vi "Write to DB.vi"() -> ()   [LabVIEW 2017]
uses:
  Type Definitions/DB Record.ctl
panel:
  in  "DB Record":T1 {"Balance" format="%.2f"; "Account" format="%05d"}
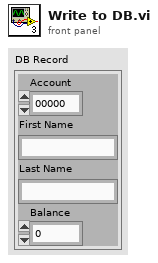
[diagram p1: front panel]
types:
  T1 = typedef "DB Record.ctl" = cluster{"Account":i32, "First Name":string, "Last Name":string, "Balance":fxp<+/-,64,35>}
  T2 = enum16{"open", "replace", "create", "open or create", "replace or create", "replace or create with confirmation"}
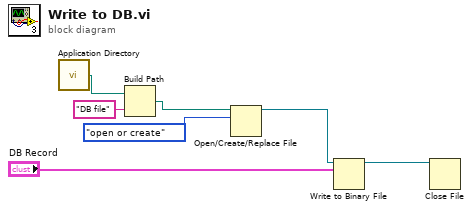
[diagram p0: block diagram]
diagram:
  n1 = call <vilib>:"Application Directory.vi"() -> ("Application Directory"=w1:path)
  n2 = Build Path(base path=w1, name or relative path="DB file") -> (appended path=w3:path)
  n3 = Open/Create/Replace File(file path (use dialog)=w3, operation (0:open)=T2."open or create") -> (refnum out=w7:refnum<file>)  [unwired: 4 in, 2 out]
  n4 = Write to Binary File(file (use dialog)=w7, data="DB Record") -> (refnum out=w5:refnum<file>)  [unwired: 4 in, 2 out]
  n5 = Close File(refnum=w5) -> ()  [unwired: 1 in, 2 out]
